vi "hmi_sistema_de_deteccion_de_fugassub.vi"() -> ()   [LabVIEW 2017]
uses:
  Control 6.ctl
  <vilib>/Utility/miscctls.llb/LVBoundsTypeDef.ctl
  <vilib>/Instr/_visa.llb/VISA Configure Serial Port (Instr).vi
  <vilib>/MakerHub/LINX/LMH-LINX.lvlib
panel:
  in  "Tab Control":enum32{"HMI", "Monitorizacion de flujo"}(tab)
  out "Boolean 2":bool
  out "FUGA 1":bool
  out "FUGA 2":bool
  out "Boolean":bool
  in  "stop 2":bool
  in  "BOMBA ON/OFF":bool
  out "FT1":bool(c317)
  out "TANQUE\n FLUIDO:AGUA":dbl(slide) scale=0.0..100.0
  in  "valvula 1":bool
  in  "valvula 2":bool
  out "TEE 02":bool
  out "TUBERIA 1IN TRAMO 02":bool(c317)
  out "TEE1":bool
  out "Multi-Segment Pipe 2":T1
  out "Multi-Segment Pipe 3":bool(c317)
  out "BOMBA 1/2 HP":bool
  out "codo90":bool
  out "Multi-Segment Pipe 4":bool(c317)
  out "FT2":bool(c317)
  out "FT 1":dbl caption="L/min"
  out "FT 2":dbl caption="L/min"
  out "67.5°":bool
  out "45°":bool
  out "22.5°":bool
  out "90°":bool
  out "SENSOR FLUJO":bool
  out "67.5° 3":bool
  out "45° 3":bool
  out "22.5° 3":bool
  out "90° 3":bool
  out "SENSOR FLUJO 3":bool
  in  "Tiempo de Muestreo":string(combo)
  in  "Jump Button 4":bool
  in  "Guardar  a Excel":bool
  in  "Rango de grafica":i16(knob) scale=0.0..100.0
  out "Flujo de entrada y salida":cluster{dbl[], dbl[]}[](graph)
  out "Tiempo de Muestreo":dbl caption="s"
  in  "Jump Button 3":bool
  in  "stop":bool
  out "Freq2":dbl
  out "Freq1":dbl
  out "Cluster":T2
  in  "Puerto":refnum<visa-resource-name>="COM3"
  in  "BaudRate":i32(ring)=10 items=["9600"=9600, "19200"=19200, "38400"=38400, "57600"=57600, "74880"=74880, "115200"=115200]
  # "PVC  1\" FLUJO: AGUA"
  # "PVC  1/2\" FLUJO: AGUA"
  # "FUGA 1"
  # "2.5 m"
  # "PVC  1/2\" FLUJO: AGUA"
  # "FUGA 2"
  # "PVC  1\" FLUJO: AGUA"
  # "6 m"
  # "MONITOREO DE SENSORES DE FLUJO YF-S201"
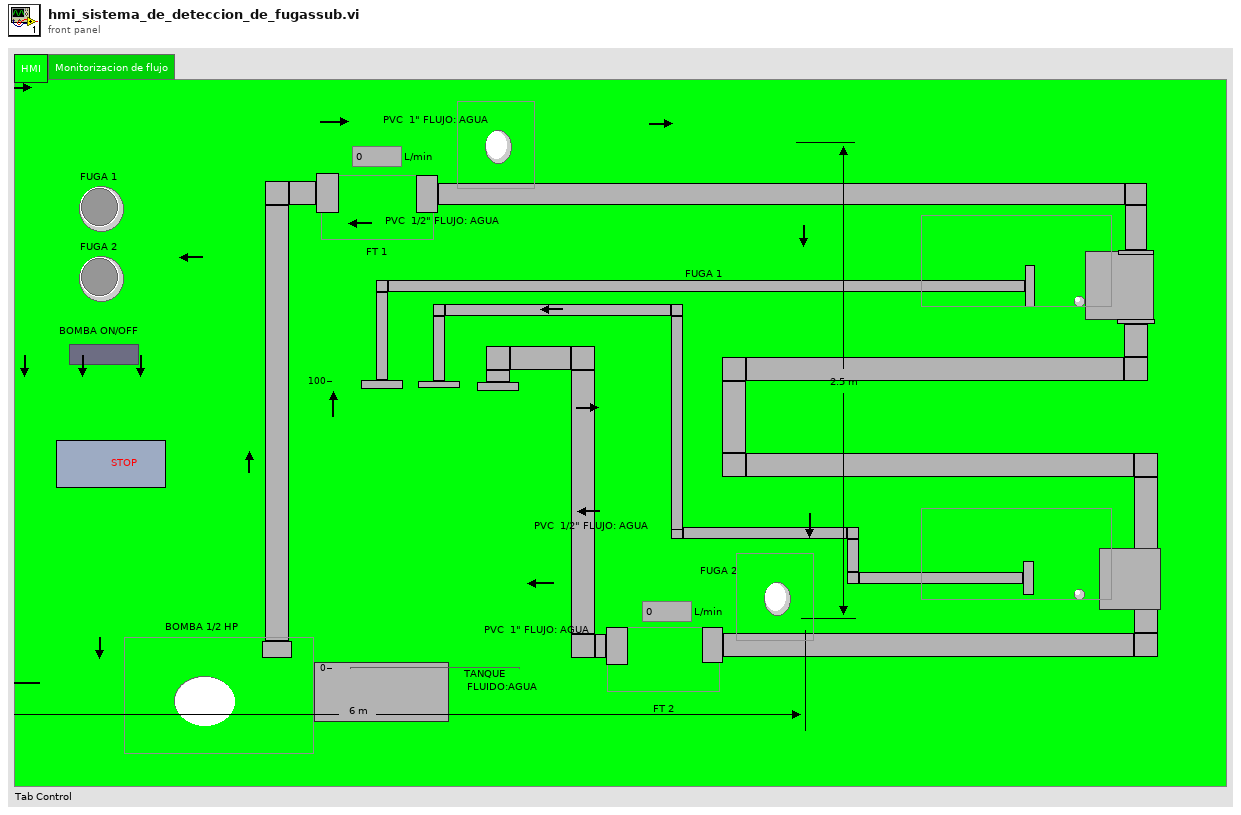
[diagram p1: front panel]
types:
  T1 = typedef "Control 6.ctl" = bool
  T2 = cluster{"FLUJO DE ENTRADA":dbl, "FLUJO DE SALIDA":dbl, "VOLUMEN 1 (L) ":dbl, "VOLUMEN 2 (L) ":dbl}
  T3 = typedef "LVBoundsTypeDef.ctl" = cluster{"Width":u32, "Height":u32}
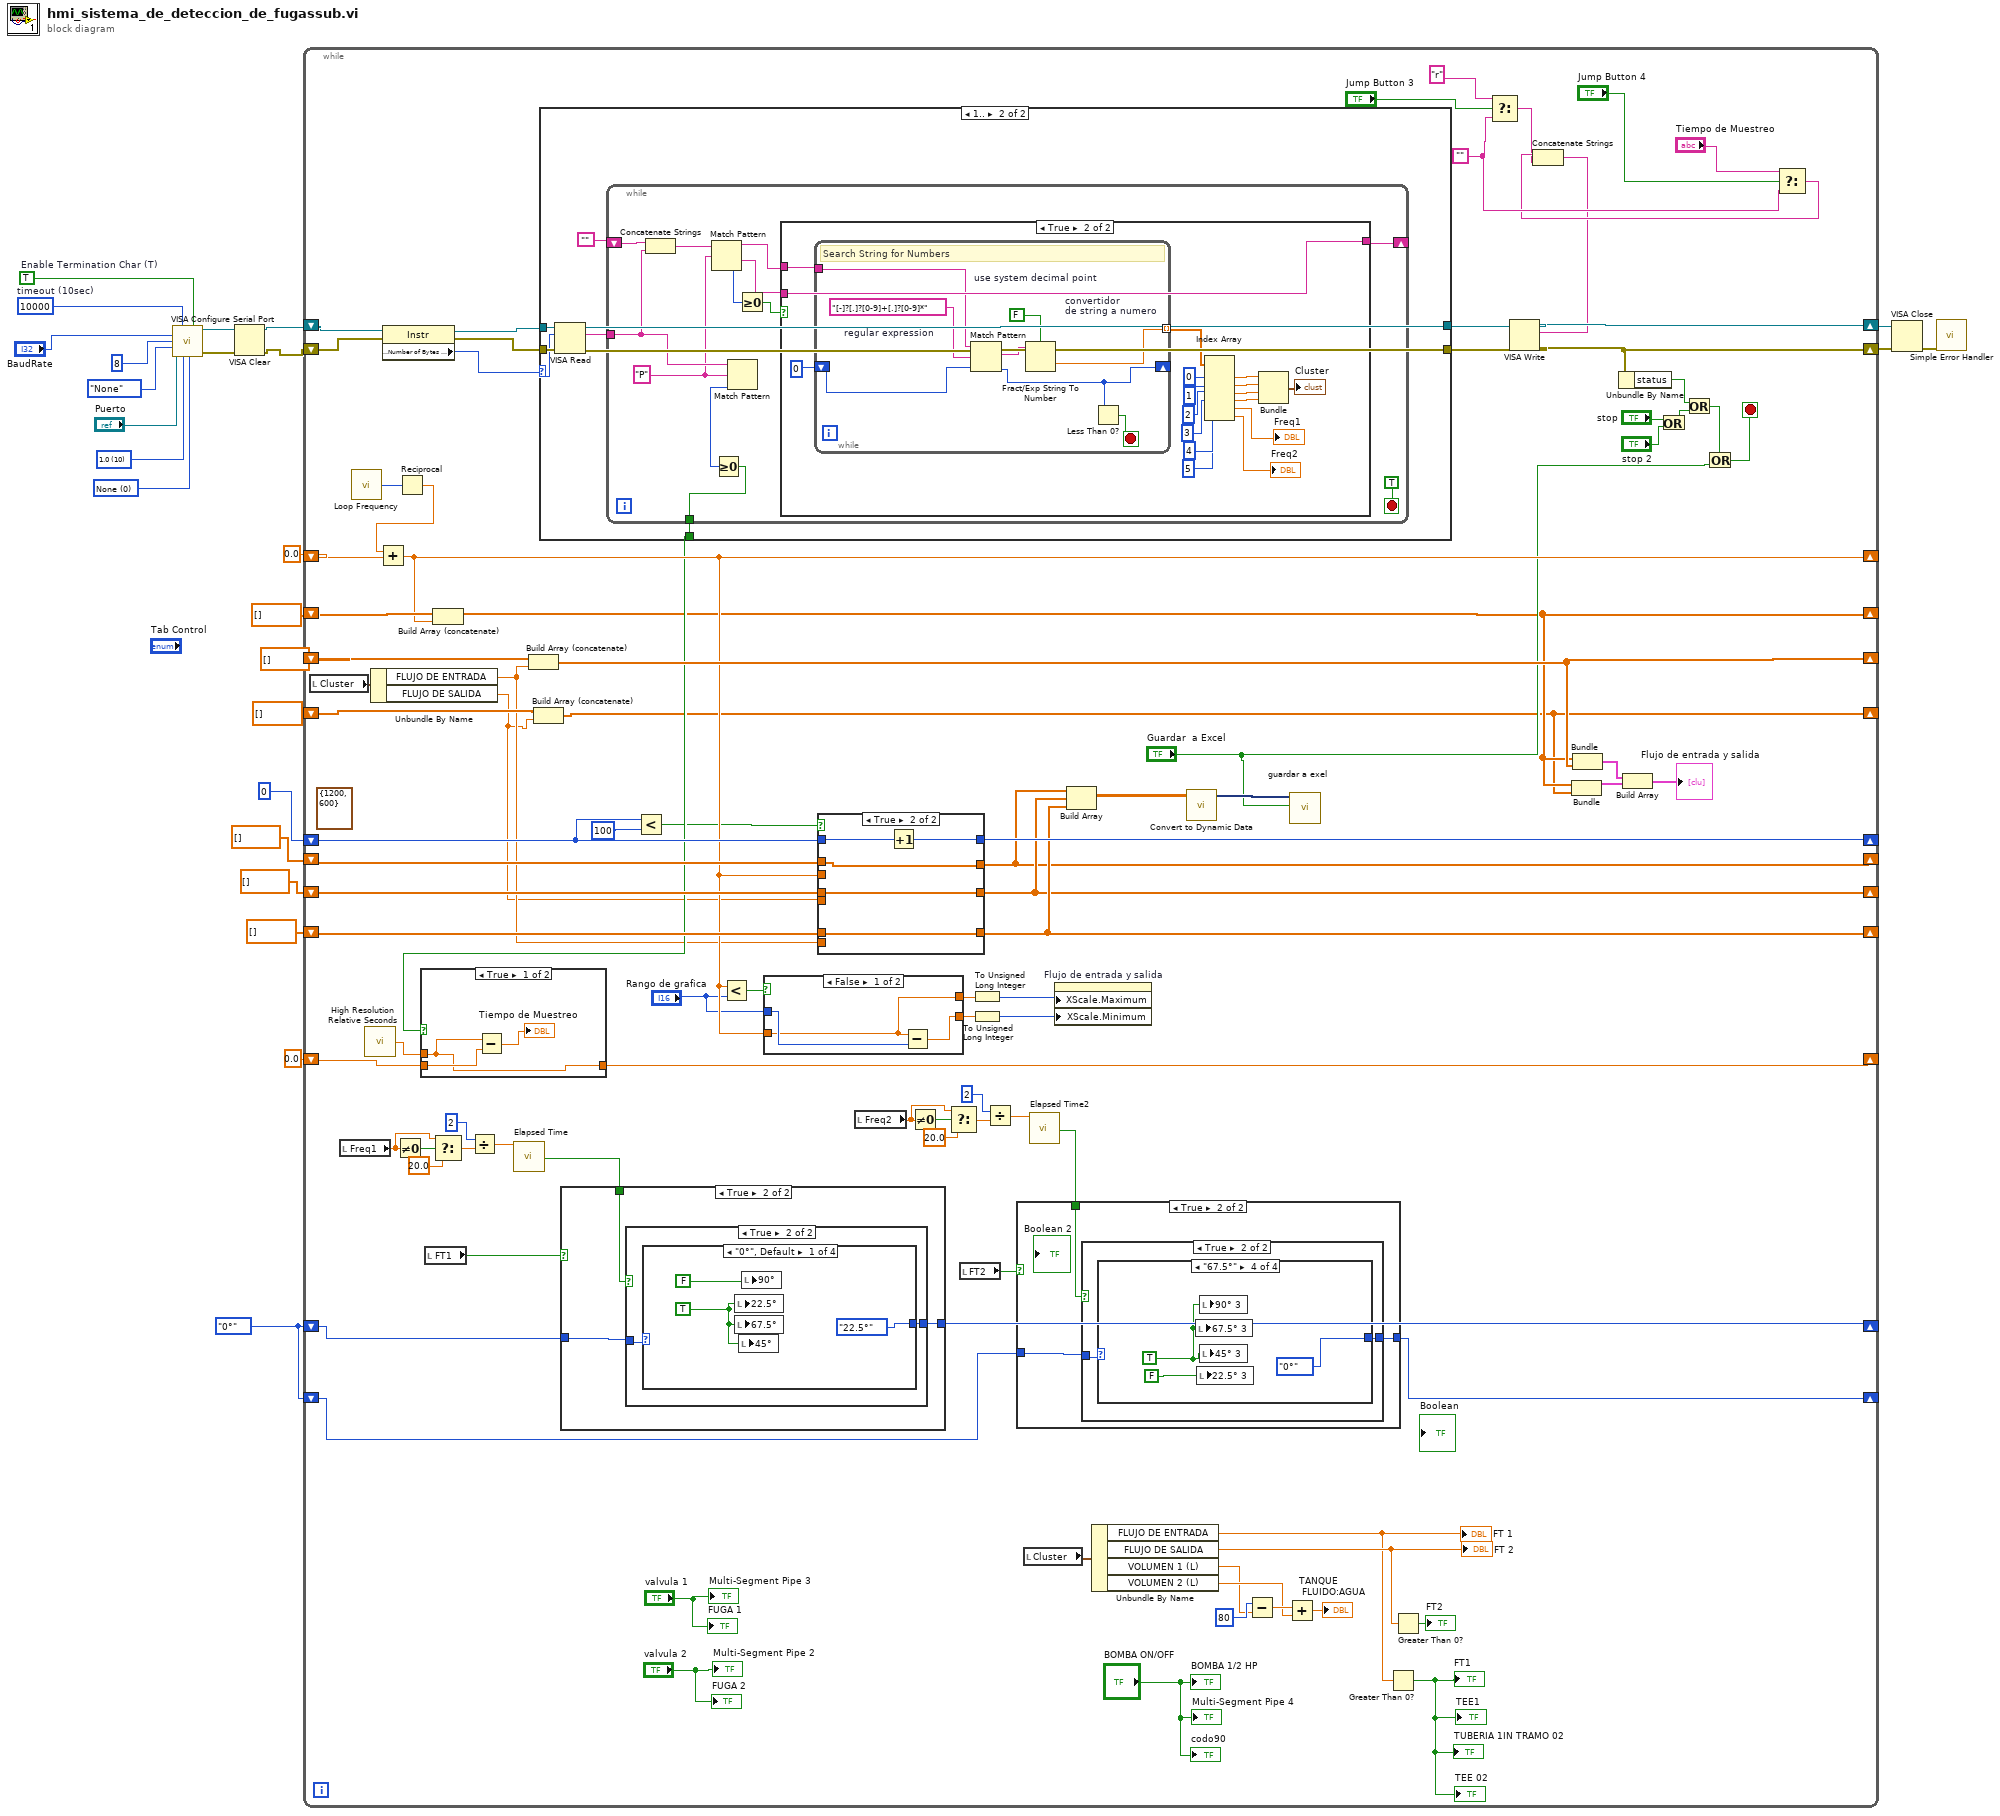
[diagram p0: block diagram]
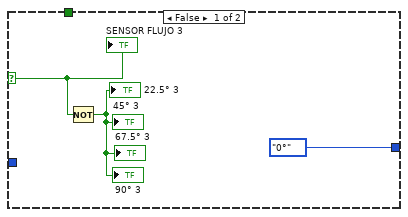
[diagram p2: hidden frame]
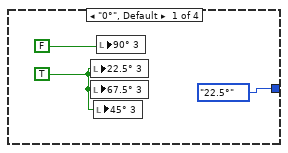
[diagram p4: hidden frame]
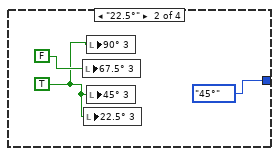
[diagram p5: hidden frame]
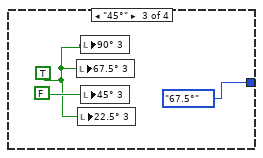
[diagram p6: hidden frame]
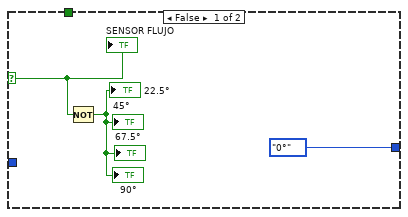
[diagram p7: hidden frame]
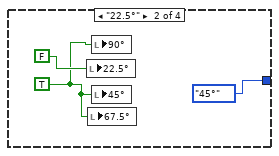
[diagram p9: hidden frame]
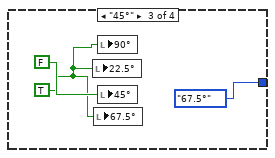
[diagram p10: hidden frame]
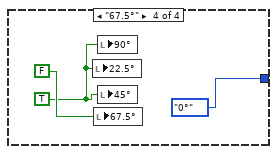
[diagram p11: hidden frame]
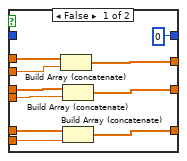
[diagram p12: hidden frame]
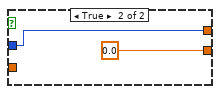
[diagram p13: hidden frame]
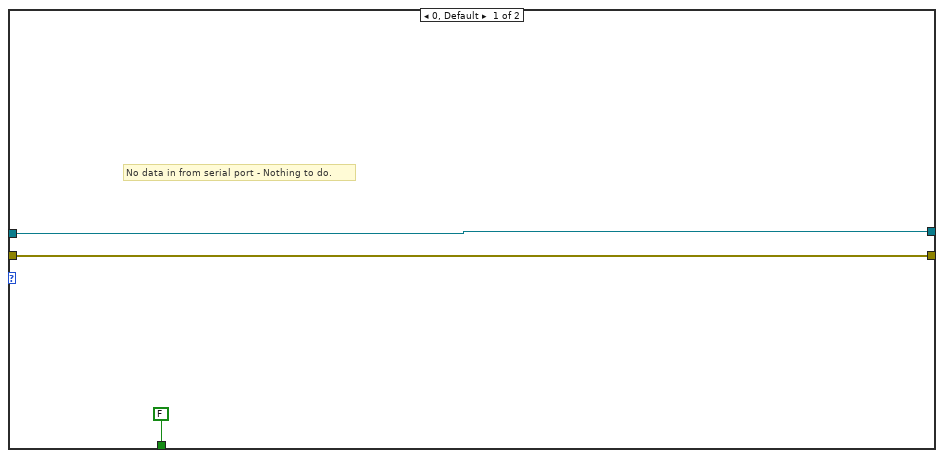
[diagram p15: hidden frame]
diagram:
  w1 = enum16{"0°", "22.5°", "45°", "67.5°"}."0°"
  w16 = u16 10 items=["1.0"=10, "1.5"=15, "2.0"=20] ("stop bits (10: 1 bit)")
  w17 = u16 0 items=["None", "XON/XOFF", "RTS/CTS", "XON/XOFF & RTS/CTS", "DTR/DSR", "XON/XOFF & DTR/DSR"] ("flow control (0:none)")
  w22 = TRUE  # Enable Termination Char (T)
  w23 = u32 10000  # timeout (10sec)
  (unwired) T3 {"Width"=1200, "Height"=600} ("Tab Control Pane Dimension")
  n1 = call-poly "VISA Configure Serial Port"("VISA resource name"="Puerto", "timeout (10sec)"=w23, "Enable Termination\nChar (T)"=w22, "baud rate (9600)"="BaudRate", "data bits (8)"=u16 8 ("Data bits (8)"), "parity (0:none)"=enum16{"None", "Odd", "Even", "Mark", "Space"}."None" ("Parity (0:none)"), "stop bits (10: 1 bit)"=w16, "flow control (0:none)"=w17) -> ("VISA resource name out"=w20:refnum<visa-resource-name>, "error out"=w21:errorcluster)  [unwired: 6 in]
  n2 = VISA Clear(VISA resource name=w20, error in (no error)=w21) -> (VISA resource name out=w19:refnum<visa-resource-name>, error out=w4:errorcluster)
  n3 = while {
    shift-right: [w66] -> _
    shift-left: dbl[] [] -> [w110]
    shift-right: [w87] -> _
    shift-left: 0.0 -> [w111]
    shift-right: [w98] -> _
    shift-left: dbl[] [] -> [w108]
    shift-right: [w65] -> _
    shift-left: dbl[] [] -> [w109]
    shift-right: [w106] -> _
    shift-left: 0.0 ("relative seconds") -> [w107]
    shift-right: [w93] -> _
    shift-left: 0 -> [w94]
    shift-right: [w88] -> _
    shift-left: dbl[] [] -> [w91]
    shift-right: [w89] -> _
    shift-left: dbl[] [] -> [w90]
    shift-right: [w86] -> _
    shift-left: dbl[] [] -> [w92]
    shift-right: [w113] -> w25
    shift-left: w4 -> [w81]
    shift-right: [w80] -> w3
    shift-left: w19 -> [w118]
    shift-right: [w51] -> _
    shift-left: w1 -> [w50]
    shift-right: [w31] -> _
    shift-left: w1 -> [w40]
    stop <- w97 stop-if-true
    w79 = ""
    n4 = local read "Cluster"() -> (w64:T2)
    n5 = local read "Freq1"() -> (w48:dbl)
    n6 = call <vilib>:"Loop Frequency.vi"() -> ("Loop Rate (Hz)"=w101:u32)
    n7 = call <vilib>:"High Resolution Relative Seconds.vi"() -> ("relative seconds"=w102:dbl)
    n8 = Unbundle By Name(w64) -> ("FLUJO DE ENTRADA"=w63:dbl, "FLUJO DE SALIDA"=w62:dbl)
    n9 = property class="Instr"(reference=w118, error in=w81) -> (reference out=w120:refnum<visa-resource-name>, error out=w119:errorcluster, "Serial Settings:Number of Bytes at Serial Port"=w117:u32)
    n10 = Not Equal To 0?(x=w48) -> (x != 0?=w49:bool)
    n11 = Reciprocal(x=w101) -> (1/x=w105:dbl)
    n12 = Add(x=w105, y=w111) -> (x+y=w87:dbl)
    n13 = local read "FT1"() -> (w52:bool)
    n14 = Build Array (concatenate)(w110, w87) -> (w66:dbl[])
    n15 = Select(t=w48, s=w49, f=20.0) -> (s? t:f=w46:dbl)
    n16 = Divide(x=i8 2, y=w46) -> (x/y=w45:dbl)
    n17 = call "Elapsed Time"("Time Target (s)"=w45) -> ("Time has Elapsed"=w43:bool)  [unwired: 11 in, 7 out]
    n18 = Build Array (concatenate)(w108, w63) -> (w98:dbl[])
    n19 = Build Array (concatenate)(w109, w62) -> (w65:dbl[])
    n20 = case shown="1.." w117 {
      selector: w117 -> [_ w193]
      tunnel: [w188 w197] -> w114
      tunnel: [w189 w196] -> w115
      tunnel: w120 -> [w189 w195]
      tunnel: w119 -> [w188 w194]
      tunnel: [FALSE w191] -> w82
      frame 0, Default {
        # "No data in from serial port - Nothing to do."
      }
      frame 1.. {
        n21 = VISA Read(VISA resource name=w195, byte count=w193, error in (no error)=w194) -> (VISA resource name out=w196:refnum<visa-resource-name>, read buffer=w192:string, error out=w197:errorcluster)  [unwired: 1 out]
        n22 = while {
          tunnel: w192 -> [w202]
          tunnel: [w200] -> w191
          shift-right: [w205] -> _
          shift-left: "" -> [w209]
          stop <- TRUE stop-if-true
          w199 = "P" ("regular expression")
          n23 = Concatenate Strings(w209, w202) -> (w204:string)
          n24 = Match Pattern(string=w204, regular expression=w199) -> (before substring=w203:string, after substring=w206:string, offset past match=w208:i32)  [unwired: 1 in, 1 out]
          n25 = Match Pattern(string=w202, regular expression=w199) -> (offset past match=w201:i32)  [unwired: 1 in, 3 out]
          n26 = Greater Or Equal To 0?(x=w201) -> (x >= 0?=w200:bool)
          n27 = Greater Or Equal To 0?(x=w208) -> (x >= 0?=w207:bool)
          n28 = case shown="True" w207 {
            tunnel: w206 -> [_ w227]
            tunnel: [w210 w227] -> w205
            tunnel: w203 -> [w210 w225]
            frame False {
            }
            frame True {
              n29 = while {
                shift-left: 0 -> [w233]
                shift-right: [w230] -> _
                tunnel: [w235] -> w222 mode=indexing
                tunnel: w225 -> [w228]
                stop <- w234 stop-if-true
                w232 = FALSE  # use system decimal point
                w229 = "[-]?[.]?[0-9]+[.]?[0-9]*"  # regular expression
                # "Search String for Numbers"
                n30 = Match Pattern(string=w228, regular expression=w229, offset (0)=w233) -> (match substring=w231:string, offset past match=w230:i32)  [unwired: 2 out]
                n31 = Fract/Exp String To Number "convertidor\nde string a numero"(use system decimal point (T)=w232, string=w231) -> (number=w235:dbl)  [unwired: 2 in, 1 out]
                n32 = Less Than 0?(x=w230) -> (x < 0?=w234:bool)
              }
              n33 = Index Array(array=w222, index #1=0 ("index"), index #2=1 ("index"), index #3=2 ("index"), index #4=3 ("index"), index #5=4 ("index"), index #6=5 ("index")) -> (element #1=w217:dbl, element #2=w216:dbl, element #3=w214:dbl, element #4=w215:dbl, element #5=→"Freq1":dbl, element #6=→"Freq2":dbl)
              n34 = Bundle(w217, w216, w214, w215) -> (→"Cluster":cluster{dbl, dbl, dbl, dbl})  [unwired: 1 in]
            }
          }
        }
      }
    }
    n35 = case shown="True" w82 {
      tunnel: w107 -> [w185 w186]
      tunnel: w102 -> [w183 _]
      tunnel: [w183 w186] -> w106
      frame True {
        n36 = Subtract(x=w183, y=w185) -> (x-y=→"Tiempo de Muestreo":dbl)
      }
      frame False {
      }
    }
    n37 = case shown="True" w52 {
      selector: w52 -> [w144 _]
      tunnel: w50 -> [_ w147]
      tunnel: [enum16{"0°", "22.5°", "45°", "67.5°"}."0°" w146] -> w51
      tunnel: w43 -> [_ w145]
      frame False {
        n38 = Not(x=w144) -> (.not. x?=→"90°" →"22.5°" →"45°" →"67.5°":bool)
        "SENSOR FLUJO" <- w144
      }
      frame True {
        n39 = case shown="True" w145 {
          tunnel: w147 -> [w148 w150]
          tunnel: [w148 w149] -> w146
          frame False {
          }
          frame True {
            n40 = case shown="\"0°\", Default" w150 {
              tunnel: [enum16{"0°", "22.5°", "45°", "67.5°"}."22.5°" enum16{"0°", "22.5°", "45°", "67.5°"}."45°" enum16{"0°", "22.5°", "45°", "67.5°"}."67.5°" enum16{"0°", "22.5°", "45°", "67.5°"}."0°"] -> w149
              frame "0°", Default {
                w151 = TRUE
                n41 = local write "22.5°"(w151) -> ()
                n42 = local write "67.5°"(w151) -> ()
                n43 = local write "45°"(w151) -> ()
                n44 = local write "90°"(FALSE) -> ()
              }
              frame "22.5°" {
                w154 = TRUE
                n45 = local write "22.5°"(FALSE) -> ()
                n46 = local write "67.5°"(w154) -> ()
                n47 = local write "90°"(w154) -> ()
                n48 = local write "45°"(w154) -> ()
              }
              frame "45°" {
                w157 = TRUE
                n49 = local write "22.5°"(w157) -> ()
                n50 = local write "67.5°"(w157) -> ()
                n51 = local write "90°"(w157) -> ()
                n52 = local write "45°"(FALSE) -> ()
              }
              frame "67.5°" {
                w160 = TRUE
                n53 = local write "22.5°"(w160) -> ()
                n54 = local write "67.5°"(FALSE) -> ()
                n55 = local write "90°"(w160) -> ()
                n56 = local write "45°"(w160) -> ()
              }
            }
          }
        }
      }
    }
    n57 = Less?(x=w94, y=u32 100) -> (x < y?=w67:bool)
    n58 = Less?(x=w87, y="Rango de grafica") -> (x < y?=w100:bool)
    n59 = case shown="False" w100 {
      tunnel: "Rango de grafica" -> [w179 w181]
      tunnel: [w178 w181] -> w72
      tunnel: [w180 0.0] -> w70
      tunnel: w87 -> [w178 _]
      frame False {
        n60 = Subtract(x=w178, y=w179) -> (x-y=w180:dbl)
      }
      frame True {
      }
    }
    n61 = case shown="True" w67 {
      tunnel: w94 -> [_ w177]
      tunnel: [u32 0 w176] -> w93
      tunnel: w92 -> [w171 w173]
      tunnel: w62 -> [w169 _]
      tunnel: [w172 w175] -> w88
      tunnel: w91 -> [w170 w175]
      tunnel: w63 -> [w167 _]
      tunnel: w90 -> [w168 w174]
      tunnel: [w166 w174] -> w89
      tunnel: [w165 w173] -> w86
      tunnel: w87 -> [w164 _]
      frame False {
        n62 = Build Array (concatenate)(w171, w164) -> (w165:dbl[])
        n63 = Build Array (concatenate)(w170, w169) -> (w172:dbl[])
        n64 = Build Array (concatenate)(w168, w167) -> (w166:dbl[])
      }
      frame True {
        n65 = Increment(x=w177) -> (x+1=w176:u32)
      }
    }
    n66 = local read "Freq2"() -> (w38:dbl)
    n67 = Not Equal To 0?(x=w38) -> (x != 0?=w39:bool)
    n68 = Select(t=w38, s=w39, f=20.0) -> (s? t:f=w36:dbl)
    n69 = local read "FT2"() -> (w32:bool)
    n70 = To Unsigned Long Integer(number=w72) -> (unsigned 32bit integer=w71:u32)
    n71 = To Unsigned Long Integer(number=w70) -> (unsigned 32bit integer=w69:u32)
    n72 = Divide(x=i8 2, y=w36) -> (x/y=w35:dbl)
    n73 = local read "Cluster"() -> (w54:T2)
    n74 = call "Elapsed Time2"("Time Target (s)"=w35) -> ("Time has Elapsed"=w33:bool)  [unwired: 11 in, 7 out]
    n75 = case shown="True" w32 {
      selector: w32 -> [w123 _]
      tunnel: w40 -> [_ w126]
      tunnel: [enum16{"0°", "22.5°", "45°", "67.5°"}."0°" w125] -> w31
      tunnel: w33 -> [_ w124]
      frame False {
        n76 = Not(x=w123) -> (.not. x?=→"90° 3" →"22.5° 3" →"45° 3" →"67.5° 3":bool)
        "SENSOR FLUJO 3" <- w123
      }
      frame True {
        n77 = case shown="True" w124 {
          tunnel: w126 -> [w127 w129]
          tunnel: [w127 w128] -> w125
          frame False {
          }
          frame True {
            n78 = case shown="\"67.5°\"" w129 {
              tunnel: [enum16{"0°", "22.5°", "45°", "67.5°"}."22.5°" enum16{"0°", "22.5°", "45°", "67.5°"}."45°" enum16{"0°", "22.5°", "45°", "67.5°"}."67.5°" enum16{"0°", "22.5°", "45°", "67.5°"}."0°"] -> w128
              frame "0°", Default {
                w130 = TRUE
                n79 = local write "22.5° 3"(w130) -> ()
                n80 = local write "67.5° 3"(w130) -> ()
                n81 = local write "45° 3"(w130) -> ()
                n82 = local write "90° 3"(FALSE) -> ()
              }
              frame "22.5°" {
                w133 = TRUE
                n83 = local write "67.5° 3"(FALSE) -> ()
                n84 = local write "22.5° 3"(w133) -> ()
                n85 = local write "90° 3"(w133) -> ()
                n86 = local write "45° 3"(w133) -> ()
              }
              frame "45°" {
                w136 = TRUE
                n87 = local write "67.5° 3"(w136) -> ()
                n88 = local write "22.5° 3"(w136) -> ()
                n89 = local write "90° 3"(w136) -> ()
                n90 = local write "45° 3"(FALSE) -> ()
              }
              frame "67.5°" {
                w139 = TRUE
                n91 = local write "67.5° 3"(w139) -> ()
                n92 = local write "22.5° 3"(FALSE) -> ()
                n93 = local write "90° 3"(w139) -> ()
                n94 = local write "45° 3"(w139) -> ()
              }
            }
          }
        }
      }
    }
    n95 = property on="Flujo de entrada y salida" class="XYGraph (strict)"("XScale.Maximum"=w71, "XScale.Minimum"=w69) -> ()  [unwired: 2 in, 2 out]
    n96 = Build Array(w86, w88, w89) -> (w84:dbl[][])
    n97 = Unbundle By Name(w54) -> ("FLUJO DE ENTRADA"=w53:dbl, "FLUJO DE SALIDA"=w60:dbl, "VOLUMEN 1 (L)"=w29:dbl, "VOLUMEN 2 (L)"=w55:dbl)
    "FT 1" <- w53
    "FT 2" <- w60
    n98 = call "Convert to Dynamic Data"("2D Array"=w84) -> ("Dynamic Data Type"=w85:dynamicdata)  [unwired: 3 in]
    n99 = Subtract(x=80, y=w29) -> (x-y=w56:dbl)
    n100 = Add(x=w56, y=w55) -> (x+y=→"TANQUE\n FLUIDO:AGUA":dbl)
    n101 = call "guardar a exel"("Signals"=w85, "Enable"="Guardar  a Excel") -> ()  [unwired: 15 in, 3 out]
    n102 = Greater Than 0?(x=w53) -> (x > 0?=→"TUBERIA 1IN TRAMO 02" →"TEE1" →"TEE 02" →"FT1":bool)
    n103 = Greater Than 0?(x=w60) -> (x > 0?=→"FT2":bool)
    n104 = Select(t="r", s="Jump Button 3", f=w79) -> (s? t:f=w76:string)
    n105 = Bundle(w66, w65) -> (w103:cluster{dbl[], dbl[]})  [unwired: 1 in]
    n106 = Bundle(w66, w98) -> (w104:cluster{dbl[], dbl[]})  [unwired: 1 in]
    n107 = Build Array(w104, w103) -> (→"Flujo de entrada y salida":cluster{dbl[], dbl[]}[])
    n108 = Or(x="stop", y="stop 2") -> (x .or. y?=w28:bool)
    n109 = Select(t="Tiempo de Muestreo", s="Jump Button 4", f=w79) -> (s? t:f=w77:string)
    n110 = Concatenate Strings(w77, w76) -> (w74:string)
    n111 = VISA Write(VISA resource name=w115, write buffer=w74, error in (no error)=w114) -> (VISA resource name out=w80:refnum<visa-resource-name>, error out=w113:errorcluster)  [unwired: 1 out]
    n112 = Unbundle By Name(w113) -> ("status"=w116:bool)
    n113 = Or(x=w116, y=w28) -> (x .or. y?=w96:bool)
    n114 = Or(x=w96, y="Guardar  a Excel") -> (x .or. y?=w97:bool)
    "BOMBA 1/2 HP" <- "BOMBA ON/OFF"
    "codo90" <- "BOMBA ON/OFF"
    "Multi-Segment Pipe 4" <- "BOMBA ON/OFF"
    "Multi-Segment Pipe 3" <- "valvula 1"
    "Multi-Segment Pipe 2" <- "valvula 2"
    "FUGA 2" <- "valvula 2"
    "FUGA 1" <- "valvula 1"
  }
  n115 = VISA Close(VISA resource name=w3, error in (no error)=w25) -> (error out=w24:errorcluster)
  n116 = call <vilib>:"Simple Error Handler.vi"("error in (no error)"=w24) -> ()  [unwired: 4 in, 5 out]
